vi "VI Tree.vi"   [LabVIEW 2012, in "Phidget Motor Position Controller.lvlib"]
doc: "${MotorPositionController:VITreeHeader}"
uses:
  <instrlib>/Phidgets/Phidget Motor Position Controller/Phidget Motor Position Controller.lvlib
  <instrlib>/Phidgets/Phidget Motor Position Controller/Public/MotorPositionControllerStart.vi
  <instrlib>/Phidgets/Phidget Motor Position Controller/Public/MotorPositionControllerOpen.vi
  <instrlib>/Phidgets/Phidget Motor Position Controller/Public/MotorPositionControllerClose.vi
panel:
  # "(c) 2015 Phidgets Inc..  ALL RIGHTS RESERVED."
  # "SEE DIAGRAM\nFOR VI TREE."
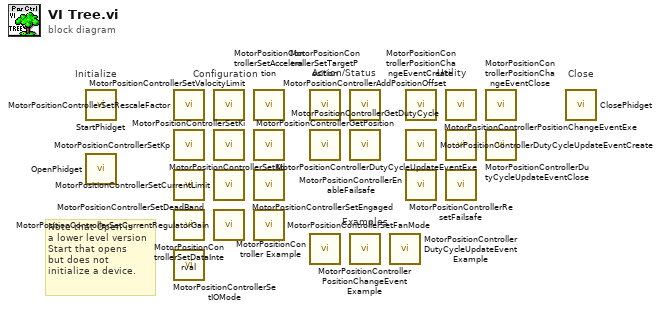
[diagram p0: block diagram]
diagram:
  # "Note that Open is\na lower level version\nStart that opens\nbut does not \ninitialize a device."
  # "Examples"
  # "Configuration"
  # "Utility"
  # "Action/Status"
  # "Close"
  # "Initialize"
  n1 = call-poly <instrlib>:"StartPhidget.vi"() -> ()  [unwired: 12 in, 4 out]
  n2 = call-poly <instrlib>:"OpenPhidget.vi"() -> ()  [unwired: 8 in, 4 out]
  n3 = call <instrlib>:"MotorPositionControllerSetRescaleFactor.vi"() -> ()  [unwired: 9 in, 2 out]
  n4 = call <instrlib>:"MotorPositionControllerSetKp.vi"() -> ()  [unwired: 9 in, 2 out]
  n5 = call <instrlib>:"MotorPositionControllerSetDeadBand.vi"() -> ()  [unwired: 9 in, 2 out]
  n6 = call <instrlib>:"MotorPositionControllerSetDataInterval.vi"() -> ()  [unwired: 9 in, 2 out]
  n7 = call <instrlib>:"MotorPositionControllerSetIOMode.vi"() -> ()  [unwired: 9 in, 2 out]
  n8 = call <instrlib>:"MotorPositionControllerSetValocityLimit.vi"() -> ()  [unwired: 9 in, 2 out]
  n9 = call <instrlib>:"MotorPositionControllerSetKi.vi"() -> ()  [unwired: 9 in, 2 out]
  n10 = call <instrlib>:"MotorPositionControllerSetCurrentLimit.vi"() -> ()  [unwired: 9 in, 2 out]
  n11 = call <instrlib>:"MotorPositionControllerSetCurrentRegulatorGain.vi"() -> ()  [unwired: 9 in, 2 out]
  n12 = call <instrlib>:"MotorPositionControllerSetAcceleration.vi"() -> ()  [unwired: 9 in, 2 out]
  n13 = call <instrlib>:"MotorPositionControllerSetKd.vi"() -> ()  [unwired: 9 in, 2 out]
  n14 = call <instrlib>:"MotorPositionControllerSetEngaged.vi"() -> ()  [unwired: 9 in, 2 out]
  n15 = call <instrlib>:"MotorPositionControllerSetFanMode.vi"() -> ()  [unwired: 9 in, 2 out]
  n16 = call <instrlib>:"MotorPositionControllerSetTargetPosition.vi"() -> ()  [unwired: 9 in, 2 out]
  n17 = call <instrlib>:"MotorPositionControllerGetPosition.vi"() -> ()  [unwired: 8 in, 3 out]
  n18 = call <instrlib>:"MotorPositionController Example.vi"() -> ()  [unwired: 12 in]
  n19 = call <instrlib>:"MotorPositionControllerAddPositionOffset.vi"() -> ()  [unwired: 9 in, 2 out]
  n20 = call <instrlib>:"MotorPositionControllerGetDutyCycle.vi"() -> ()  [unwired: 8 in, 3 out]
  n21 = call <instrlib>:"MotorPositionController PositionChangeEvent Example.vi"() -> ()  [unwired: 12 in]
  n22 = call <instrlib>:"MotorPositionController DutyCycleUpdateEvent Example.vi"() -> ()  [unwired: 12 in]
  n23 = call <instrlib>:"MotorPositionControllerPositionChangeEventCreate.vi"() -> ()  [unwired: 9 in, 3 out]
  n24 = call <instrlib>:"MotorPositionControllerDutyCycleUpdateEventCreate.vi"() -> ()  [unwired: 9 in, 3 out]
  n25 = call <instrlib>:"MotorPositionControllerEnableFailsafe.vi"() -> ()  [unwired: 9 in, 2 out]
  n26 = call <instrlib>:"MotorPositionControllerPositionChangeEventExe.vi"() -> ()  [unwired: 5 in, 7 out]
  n27 = call <instrlib>:"MotorPositionControllerDutyCycleUpdateEventExe.vi"() -> ()  [unwired: 5 in, 7 out]
  n28 = call <instrlib>:"MotorPositionControllerResetFailsafe.vi"() -> ()  [unwired: 9 in, 2 out]
  n29 = call <instrlib>:"MotorPositionControllerPositionChangeEventClose.vi"() -> ()  [unwired: 10 in, 2 out]
  n30 = call <instrlib>:"MotorPositionControllerDutyCycleUpdateEventClose.vi"() -> ()  [unwired: 10 in, 2 out]
  n31 = call-poly <instrlib>:"ClosePhidget.vi"() -> ()  [unwired: 11 in, 1 out]
